vi "C3 - Read.vi"(8 "error in":errorcluster, 11 "TSM Context Global Access in":refnum<class "TSM Context Data Access.lvclass">) -> (0 "error out":errorcluster, 2 "C3":dbl[][](array[numeric]), 3 "TSM Context Global Access out":refnum<class "TSM Context Data Access.lvclass">)   [LabVIEW 2019, in "TSM Context Data Access.lvclass"]
uses:
  TSM Context Data Access.lvclass
  TSM Context Data Access.lvclass/TSM Context Data Access.ctl
  <vilib>/NI_TestStand_SemiconductorModule/NI_TestStand_Semiconductor_Module.lvlibp
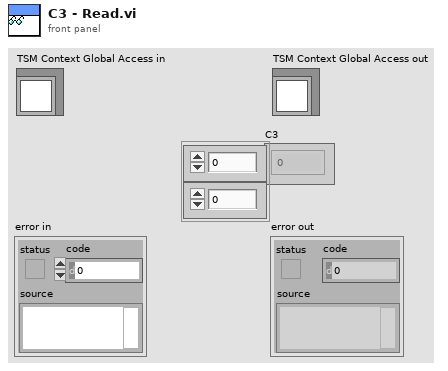
[diagram p1: front panel]
types:
  T1 = typedef "NI_TestStand_Semiconductor_Module.lvlibp/SemiconductorModuleContext.ctl" = refnum<k7>
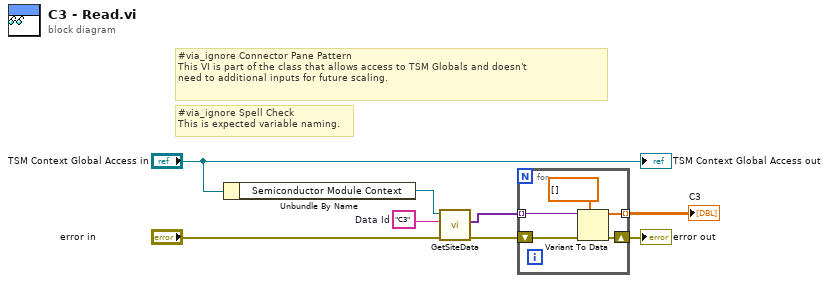
[diagram p0: block diagram]
diagram:
  w4 = "C3"  # Data Id
  # "#via_ignore Spell Check\nThis is expected variable naming."
  # "#via_ignore Connector Pane Pattern \nThis VI is part of the class that allows access to TSM Globals and doesn't \nneed to additional inputs for future scaling."
  n1 = Unbundle By Name("TSM Context Global Access in") -> ("Semiconductor Module Context"=w5:T1)
  n2 = call <vilib>:"GetSiteData.vi"("error in (no error)"="error in", "Data Id"=w4, "Semiconductor Module Context"=w5) -> ("error out"=w6:errorcluster, "Site Data"=w1:variant[])  [unwired: 6 in, 1 out]
  n3 = for {
    shift-right: [w12] -> w3
    shift-left: w6 -> [w13]
    tunnel: w1 -> [w11] mode=indexing
    tunnel: [w10] -> w2 mode=indexing
    n4 = Variant To Data(error in=w13, type=dbl[] [], Variant=w11) -> (data=w10:dbl[], error out=w12:errorcluster)
  }
  "error out" <- w3
  "C3" <- w2
  "TSM Context Global Access out" <- "TSM Context Global Access in"
